vi "UpdateVariablesTCGroupView.vi"(8 "error in (no error)":errorcluster, 11 "VMUI in":refnum<class "VMUI.lvclass">) -> (0 "error out":errorcluster, 3 "VMUI out":refnum<class "VMUI.lvclass">)   [LabVIEW 2013, in "VMUI.lvclass"]
uses:
  VMUI.lvclass
  VariableManager/VariableManager.lvclass
  VariableGroup/VariableGroup.lvclass
  API/VariableManagerAPI.lvlib
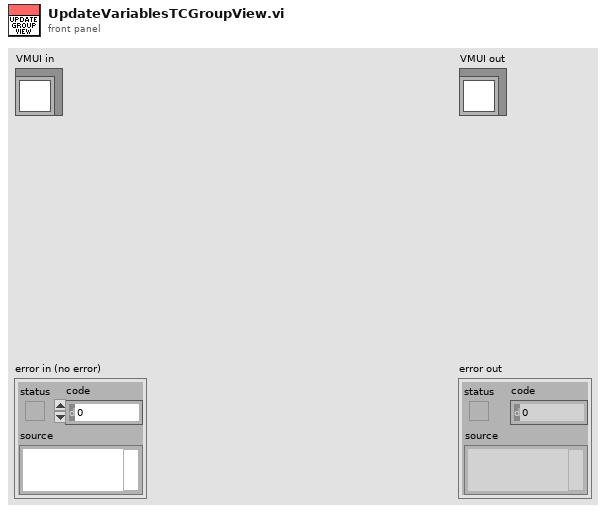
[diagram p1: front panel]
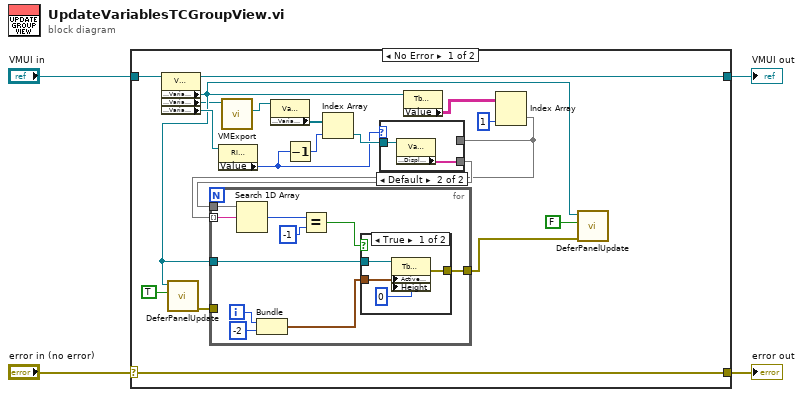
[diagram p0: block diagram]
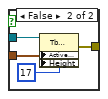
[diagram p3: hidden frame]
diagram:
  n1 = case shown="No Error" "error in (no error)" {
    selector: "error in (no error)" -> [w23 w46]
    tunnel: [w23 w46] -> w3
    tunnel: [w21 w45] -> w1
    tunnel: "VMUI in" -> [w22 w45]
    frame No Error {
      n2 = property class="VMUI.lvclass"(reference=w22) -> (reference out=w21:refnum<class "VMUI.lvclass">, "Accessors:VariablesTCRef"=w10:refnum<vi>, "Accessors:VariableManagerRef"=w8:refnum<vi>, "Accessors:VariableGroupRingRef"=w20:refnum<vi>)  [unwired: 1 in, 1 out]
      n3 = call "DeferPanelUpdate.vi"("Defer Panel Updates"=TRUE, "GObjectRefIn"=w10) -> ("error out"=w6:errorcluster)  [unwired: 9 in]
      n4 = property class="Ring (strict)"(reference=w20) -> ("Value"=w15:u16)  [unwired: 1 in, 2 out]
      n5 = call "VMExport.vi"("VariableManagerRef in"=w8) -> ("VariableManagerExportCopy"=w7:refnum<class "VariableManager.lvclass">)  [unwired: 8 in, 2 out]
      n6 = property class="VariableManager.lvclass"(reference=w7) -> ("Accessors:VariableGroups"=w9:refnum<class "VariableGroup.lvclass">[])  [unwired: 1 in, 2 out]
      n7 = Decrement(x=w15) -> (x-1=w14:u16)
      n8 = Index Array(array=w9, index=w14) -> (element=w19:refnum<class "VariableGroup.lvclass">)
      n9 = property class="Tbl (strict)"(reference=w10) -> ("Value"=w18:string[][])  [unwired: 1 in, 2 out]
      n10 = Index Array(array=w18, index (col)=1 ("disabled index (col)")) -> (element=w13:string[])  [unwired: 1 in]
      n11 = case shown="Default" w15 {
        tunnel: w19 -> [_ w26]
        tunnel: [w24 w25] -> w16
        tunnel: w13 -> [w24 _]
        frame 0 {
        }
        frame Default {
          n12 = property class="VariableGroup.lvclass"(reference=w26) -> ("Accessors:DisplayList"=w25:string[])  [unwired: 1 in, 2 out]
        }
      }
      n13 = for {
        tunnel: w13 -> [w35] mode=indexing
        tunnel: w16 -> [w36]
        tunnel: w10 -> [w28]
        tunnel: w6 -> [_]
        tunnel: [w27] -> w5
        i -> [w32]
        n14 = Search 1D Array(1D array=w36, element=w35) -> (index of element=w34:i32)  [unwired: 1 in]
        n15 = Bundle(w32, "Column"=-2) -> (w30:cluster{i32, "Column":i32})  [unwired: 1 in]
        n16 = Equal?(x=w34, y=-1) -> (x = y?=w29:bool)
        n17 = case shown="True" w29 {
          tunnel: w28 -> [w40 w44]
          tunnel: w30 -> [w39 w43]
          tunnel: [w37 w41] -> w27
          frame True {
            n18 = property class="Tbl (strict)"(reference=w40, "Active Cell"=w39, "Height"=u32 0 ("Active Cell:Cell Size:Height")) -> (error out=w37:errorcluster)  [unwired: 1 in, 1 out]
          }
          frame False {
            n19 = property class="Tbl (strict)"(reference=w44, "Active Cell"=w43, "Height"=u32 17 ("Active Cell:Cell Size:Height")) -> (error out=w41:errorcluster)  [unwired: 1 in, 1 out]
          }
        }
      }
      n20 = call "DeferPanelUpdate.vi"("error in (no error)"=w5, "Defer Panel Updates"=FALSE, "GObjectRefIn"=w10) -> ()  [unwired: 8 in, 1 out]
    }
    frame Error {
    }
  }
  "error out" <- w3
  "VMUI out" <- w1
